vi "True once (SubVI).vi"(1 "Automatic":bool) -> (0 "Boolean":bool)   [LabVIEW 2014]
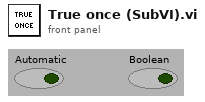
[diagram p1: front panel]
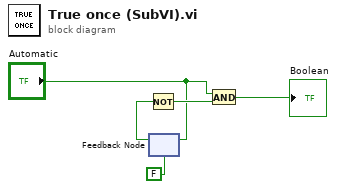
[diagram p0: block diagram]
diagram:
  n1 = feedback #1(FALSE) -> (w3:bool)
  n2 = Not(x=w3) -> (.not. x?=w4:bool)
  n3 = feedback-in #1("Automatic") -> ()
  n4 = And(x="Automatic", y=w4) -> (x .and. y?=→"Boolean":bool)
